vi "XML Reader Start Section.vi"(6 "Default Attribute Values":variant[](array[variant]), 7 "Attribute Names":string[](array[string]), 8 "error in":errorcluster, 10 "Element Name":string, 11 "XML Reader In":T1) -> (0 "error out":errorcluster, 1 "Attribute Values":variant[](array[variant]), 2 "Found?":bool, 3 "XML Reader Out":T1)   [LabVIEW 2016, in "Pathloss XML Reader.lvlib"]
uses:
  Pathloss XML Reader.lvlib
  Controls/XML Reader Data Ref.ctl
  Controls/XML Reader Data.ctl
  <vilib>/Utility/VariantDataType/VariantType.lvlib
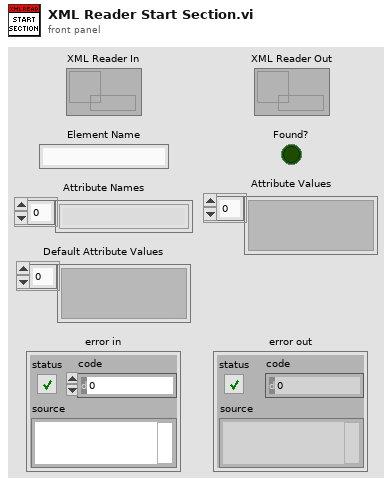
[diagram p1: front panel]
types:
  T1 = typedef "Pathloss XML Reader.lvlib/XML Reader Data Ref.ctl" = refnum<data-value>
  T2 = typedef "Pathloss XML Reader.lvlib/XML Reader Data.ctl" = cluster{"Remaining XML":string, "Section Name Stack":string[], "Section Stack":string[]}
  T3 = typedef "VariantType.lvlib/Type.ctl" = enum8{"Invalid Type", "Void", "I8", "I16", "I32", "I64", "U8", "U16", "U32", "U64", "Single Float", "Double Float", "Extended Float", "Single Complex", "Double Complex", "Extended Complex", "Enum U8", "Enum U16", "Enum U32", "Enum U64", "Single Float With Unit", "Double Float With Unit", "Extended Float With Unit", "Single Complex with Unit", "Double Complex with Unit", "Extended Complex with Unit", "Boolean", "String", "Path", "Picture", "Tag", "Array", "Cluster", "Variant", "LV Variant", "Waveform", "Timestamp", "Digital Waveform", "Digital Data", "ExpressData", "Refnum", "External Data", "VI", "Poly VI", "LabVIEW Class Instance", "Fixed Point"}
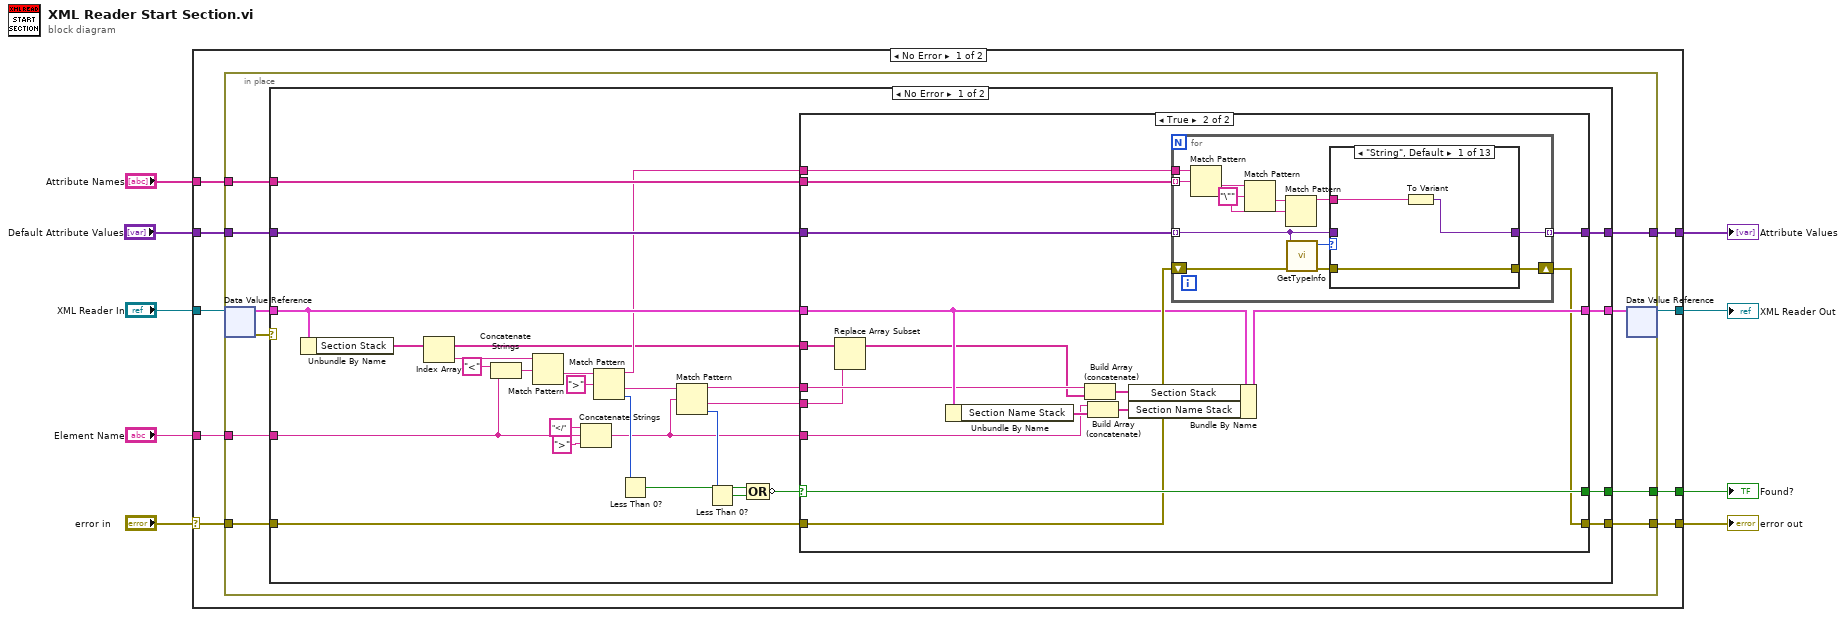
[diagram p0: block diagram]
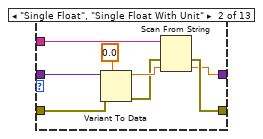
[diagram p3: hidden frame]
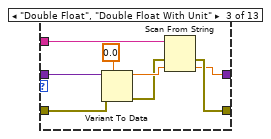
[diagram p4: hidden frame]
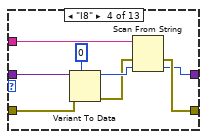
[diagram p5: hidden frame]
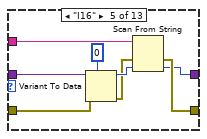
[diagram p6: hidden frame]
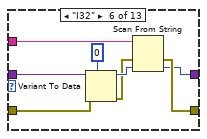
[diagram p7: hidden frame]
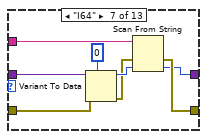
[diagram p8: hidden frame]
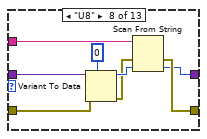
[diagram p9: hidden frame]
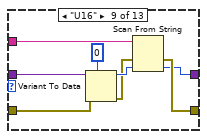
[diagram p10: hidden frame]
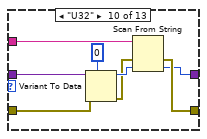
[diagram p11: hidden frame]
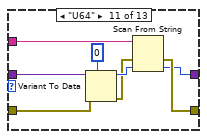
[diagram p12: hidden frame]
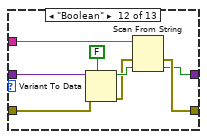
[diagram p13: hidden frame]
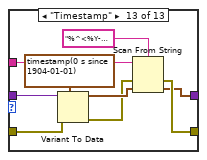
[diagram p14: hidden frame]
diagram:
  n1 = case shown="No Error" "error in" {
    selector: "error in" -> [w16 w193]
    tunnel: [w15 w193] -> w8
    tunnel: [w17 w194] -> w7
    tunnel: "XML Reader In" -> [w18 w194]
    tunnel: "Element Name" -> [w14 _]
    tunnel: "Attribute Names" -> [w13 _]
    tunnel: "Default Attribute Values" -> [w12 w192]
    tunnel: [w11 _] -> w1
    tunnel: [w10 w192] -> w2
    frame No Error {
      n2 = in-place {
        in-place-border: w16 -> [w25]
        in-place-border: [w24] -> w15
        in-place-border: w14 -> [w23]
        in-place-border: w13 -> [w22]
        in-place-border: w12 -> [w21]
        in-place-border: [w20] -> w11
        in-place-border: [w19] -> w10
        n3 = in-place-dvr #1(w18) -> (w27:T2, w28:errorcluster)
        n4 = case shown="No Error" w28 {
          selector: w28 -> [_ w190]
          tunnel: w27 -> [w46 w191]
          tunnel: [w45 w191] -> w26
          tunnel: w25 -> [w48 _]
          tunnel: [w47 w190] -> w24
          tunnel: w23 -> [w33 _]
          tunnel: w22 -> [w42 _]
          tunnel: w21 -> [w43 w189]
          tunnel: [w44 _] -> w20
          tunnel: [w41 w189] -> w19
          frame No Error {
            n5 = Unbundle By Name(w46) -> ("Section Stack"=w37:string[])
            n6 = Index Array(array=w37) -> (element=w38:string)  [unwired: 1 in]
            n7 = Concatenate Strings("<" ("string"), w33) -> (w54:string)
            n8 = Match Pattern(string=w38, regular expression=w54) -> (after substring=w53:string)  [unwired: 1 in, 3 out]
            n9 = Concatenate Strings("</" ("string"), w33, ">" ("string")) -> (w30:string)
            n10 = Match Pattern(string=w53, regular expression=">") -> (before substring=w40:string, after substring=w34:string, offset past match=w39:i32)  [unwired: 1 in, 1 out]
            n11 = Less Than 0?(x=w39) -> (x < 0?=w51:bool)
            n12 = Match Pattern(string=w34, regular expression=w30) -> (before substring=w31:string, after substring=w29:string, offset past match=w32:i32)  [unwired: 1 in, 1 out]
            n13 = Less Than 0?(x=w32) -> (x < 0?=w50:bool)
            n14 = Compound Arithmetic op=OR(w51, w50) -> (invert w49:bool)
            n15 = case shown="True" w49 {
              selector: w49 -> [w57 w75]
              tunnel: w48 -> [w58 w69]
              tunnel: [w58 w71] -> w47
              tunnel: w46 -> [w59 w68]
              tunnel: [w59 w76] -> w45
              tunnel: w40 -> [_ w73]
              tunnel: [w57 w75] -> w44
              tunnel: w43 -> [w56 w72]
              tunnel: w42 -> [_ w74]
              tunnel: [w56 w70] -> w41
              tunnel: w30 -> [_ w66]
              tunnel: w37 -> [_ w62]
              tunnel: w31 -> [_ w63]
              tunnel: w29 -> [_ w60]
              frame False {
              }
              frame True {
                n16 = Replace Array Subset(array=w62, new element=w60) -> (w61:string[])  [unwired: 1 in]
                n17 = Unbundle By Name(w68) -> ("Section Name Stack"=w67:string[])
                n18 = Build Array (concatenate)(w63, w61) -> (w64:string[])
                n19 = Build Array (concatenate)(w66, w67) -> (w65:string[])
                n20 = Bundle By Name(cluster=w68, "Section Stack"=w64, "Section Name Stack"=w65) -> (w76:T2)
                n21 = for {
                  tunnel: w73 -> [w88]
                  tunnel: w74 -> [w87] mode=indexing
                  tunnel: w72 -> [w80] mode=indexing
                  shift-right: [w78] -> w71
                  shift-left: w69 -> [w83]
                  tunnel: [w77] -> w70 mode=indexing
                  w84 = "\"" ("regular expression")
                  n22 = Match Pattern(string=w88, regular expression=w87) -> (after substring=w86:string)  [unwired: 1 in, 3 out]
                  n23 = Match Pattern(string=w86, regular expression=w84) -> (after substring=w85:string)  [unwired: 1 in, 3 out]
                  n24 = Match Pattern(string=w85, regular expression=w84) -> (before substring=w81:string)  [unwired: 1 in, 3 out]
                  n25 = call <vilib>:"GetTypeInfo.vi"("error in (no error)"=w83, "Variant"=w80) -> ("error out"=w79:errorcluster, "Type Enum"=w82:T3)  [unwired: 5 in, 3 out]
                  n26 = case shown="\"String\", Default" w82 {
                    tunnel: w81 -> [w90 w99 w107 w115 w123 w131 w139 w147 w155 w163 w171 w179 w188]
                    tunnel: w80 -> [_ w98 w106 w114 w122 w130 w138 w146 w154 w162 w170 w178 w187]
                    tunnel: w79 -> [w91 w97 w105 w113 w121 w129 w137 w145 w153 w161 w169 w177 w186]
                    tunnel: [w91 w94 w102 w110 w118 w126 w134 w142 w150 w158 w166 w174 w183] -> w78
                    tunnel: [w89 w92 w100 w108 w116 w124 w132 w140 w148 w156 w164 w172 w181] -> w77
                    frame "String", Default {
                      n27 = To Variant(anything=w90) -> (Variant=w89:variant)
                    }
                    frame "Single Float", "Single Float With Unit" {
                      n28 = Variant To Data(error in=w97, type=sgl 0.0, Variant=w98) -> (data=w96:sgl, error out=w95:errorcluster)
                      n29 = Scan From String(input string=w99, error in=w95, default 1=w96) -> (error out=w94:errorcluster, output 1=w92:sgl)  [unwired: 2 in, 2 out]
                    }
                    frame "Double Float", "Double Float With Unit" {
                      n30 = Variant To Data(error in=w105, type=0.0, Variant=w106) -> (data=w104:dbl, error out=w103:errorcluster)
                      n31 = Scan From String(input string=w107, error in=w103, default 1=w104) -> (error out=w102:errorcluster, output 1=w100:dbl)  [unwired: 2 in, 2 out]
                    }
                    frame "I8" {
                      n32 = Variant To Data(error in=w113, type=i8 0, Variant=w114) -> (data=w112:i8, error out=w111:errorcluster)
                      n33 = Scan From String(input string=w115, error in=w111, default 1=w112) -> (error out=w110:errorcluster, output 1=w108:i8)  [unwired: 2 in, 2 out]
                    }
                    frame "I16" {
                      n34 = Variant To Data(error in=w121, type=i16 0, Variant=w122) -> (data=w120:i16, error out=w119:errorcluster)
                      n35 = Scan From String(input string=w123, error in=w119, default 1=w120) -> (error out=w118:errorcluster, output 1=w116:i16)  [unwired: 2 in, 2 out]
                    }
                    frame "I32" {
                      n36 = Variant To Data(error in=w129, type=0, Variant=w130) -> (data=w128:i32, error out=w127:errorcluster)
                      n37 = Scan From String(input string=w131, error in=w127, default 1=w128) -> (error out=w126:errorcluster, output 1=w124:i32)  [unwired: 2 in, 2 out]
                    }
                    frame "I64" {
                      n38 = Variant To Data(error in=w137, type=i64 0, Variant=w138) -> (data=w136:i64, error out=w135:errorcluster)
                      n39 = Scan From String(input string=w139, error in=w135, default 1=w136) -> (error out=w134:errorcluster, output 1=w132:i64)  [unwired: 2 in, 2 out]
                    }
                    frame "U8" {
                      n40 = Variant To Data(error in=w145, type=u8 0, Variant=w146) -> (data=w144:u8, error out=w143:errorcluster)
                      n41 = Scan From String(input string=w147, error in=w143, default 1=w144) -> (error out=w142:errorcluster, output 1=w140:u8)  [unwired: 2 in, 2 out]
                    }
                    frame "U16" {
                      n42 = Variant To Data(error in=w153, type=u16 0, Variant=w154) -> (data=w152:u16, error out=w151:errorcluster)
                      n43 = Scan From String(input string=w155, error in=w151, default 1=w152) -> (error out=w150:errorcluster, output 1=w148:u16)  [unwired: 2 in, 2 out]
                    }
                    frame "U32" {
                      n44 = Variant To Data(error in=w161, type=u32 0, Variant=w162) -> (data=w160:u32, error out=w159:errorcluster)
                      n45 = Scan From String(input string=w163, error in=w159, default 1=w160) -> (error out=w158:errorcluster, output 1=w156:u32)  [unwired: 2 in, 2 out]
                    }
                    frame "U64" {
                      n46 = Variant To Data(error in=w169, type=u64 0, Variant=w170) -> (data=w168:u64, error out=w167:errorcluster)
                      n47 = Scan From String(input string=w171, error in=w167, default 1=w168) -> (error out=w166:errorcluster, output 1=w164:u64)  [unwired: 2 in, 2 out]
                    }
                    frame "Boolean" {
                      n48 = Variant To Data(error in=w177, type=FALSE, Variant=w178) -> (data=w176:bool, error out=w175:errorcluster)
                      n49 = Scan From String(input string=w179, error in=w175, default 1=w176) -> (error out=w174:errorcluster, output 1=w172:bool)  [unwired: 2 in, 2 out]
                    }
                    frame "Timestamp" {
                      n50 = Variant To Data(error in=w186, type=timestamp(0 s since 1904-01-01), Variant=w187) -> (data=w185:timestamp, error out=w184:errorcluster)
                      n51 = Scan From String(format string="%^<%Y-%m-%dT%H:%M:%S%7u%z>T" ("regular expression"), input string=w188, error in=w184, default 1=w185) -> (error out=w183:errorcluster, output 1=w181:timestamp)  [unwired: 1 in, 2 out]
                    }
                  }
                }
              }
            }
          }
          frame Error {
          }
        }
        n52 = in-place-dvr #1(w26) -> (w17:T1)  [unwired: 1 out]
      }
    }
    frame Error {
    }
  }
  "error out" <- w8
  "XML Reader Out" <- w7
  "Attribute Values" <- w2
  "Found?" <- w1
